vi "GlobalVarDrive_2.vi"() -> ()   [LabVIEW 2016]
panel:
  in  "Joystick 2 (RS Y-Axis)":dbl
  in  "Joystick 2 (RS X-Axis)":dbl
  in  "Joystick 2 (LS Y-Axis)":dbl
  in  "Joystick 2 (LS X-Axis)":dbl
  in  "Joystick 1 (RS Y-Axis)":dbl
  in  "Joystick 1 (RS X-Axis)":dbl
  in  "Joystick 1 (LS Y-Axis)":dbl
  in  "Joystick 1 (LS X-Axis)":dbl
  out "Joystick 2 (Start)":bool
  out "Joystick 2 (Back)":bool
  out "Joystick 2 (RB)":bool
  out "Joystick 2 (LB)":bool
  out "Joystick 2 (RT)":bool
  out "Joystick 2 (LT)":bool
  out "Joystick 2 (Y)":bool
  out "Joystick 2 (X)":bool
  out "Joystick 2 (B)":bool
  out "Joystick 2 (A)":bool
  out "Joystick 1 (LS Y-Axis)":bool
  out "Joystick 1 (Start)":bool
  out "Joystick 1 (Back)":bool
  out "Joystick 1 (RB)":bool
  out "Joystick 1 (LB)":bool
  out "Joystick 1 (RT)":bool
  out "Joystick 1 (LT)":bool
  out "Joystick 1 (Y)":bool
  out "Joystick 1 (X)":bool
  out "Joystick 1 (B)":bool
  out "Joystick 1 (A)":bool
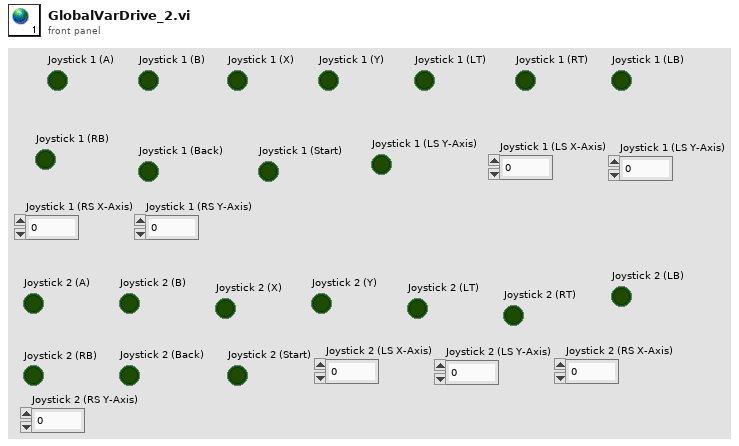
[diagram p1: front panel]
diagram:
